vi "Rolling Average.vi"(7 "Enum":enum16{"Positive Slope", "Negative Slope"}(ring), 10 "Filtered X":dbl[](array[numeric]), 11 "Subset Length":i32) -> (3 "Averaged Values":dbl[][](array[numeric]))   [LabVIEW 2018]
uses:
  <vilib>/Analysis/baseanly.llb/Mean (DBL).vi
  <vilib>/Analysis/NI_AALBase.lvlib
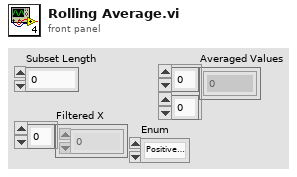
[diagram p1: front panel]
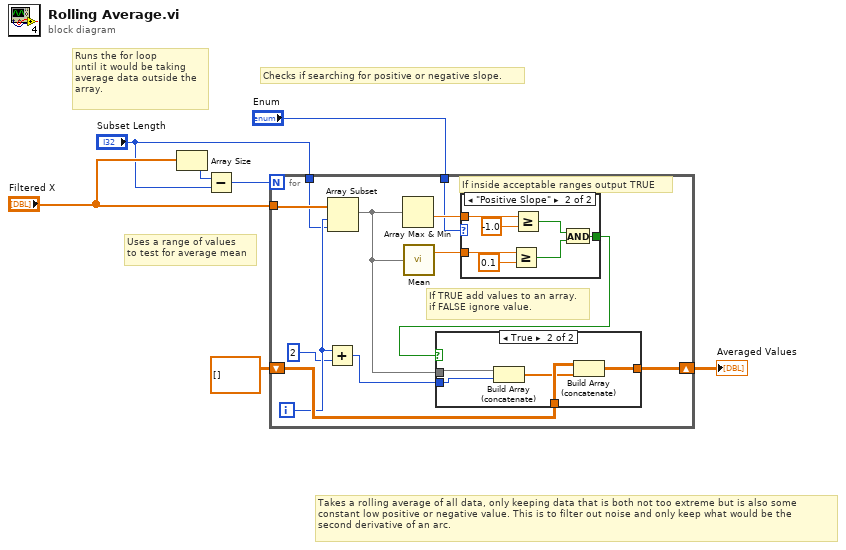
[diagram p0: block diagram]
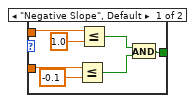
[diagram p2: hidden frame]
diagram:
  # "Uses a range of values\nto test for average mean"
  # "Checks if searching for positive or negative slope."
  # "Runs the for loop\nuntil it would be taking \naverage data outside the \narray."
  # "Takes a rolling average of all data, only keeping data that is both not too extreme but is also some\nconstant low positive or negative value. This is to filter out noise and only keep what would be the \nsecond derivative of an arc."
  n1 = Array Size(array="Filtered X") -> (size(s)=w3:i32)
  n2 = Subtract(x=w3, y="Subset Length") -> (x-y=w4:i32)
  n3 = for {
    N: w4 -> [_]
    tunnel: "Filtered X" -> [w19]
    shift-right: [w15] -> w7
    shift-left: dbl[][] [] -> [w14]
    tunnel: "Subset Length" -> [w10]
    tunnel: "Enum" -> [w9]
    i -> [w13]
    # "If TRUE add values to an array.\nif FALSE ignore value."
    # "If inside acceptable ranges output TRUE"
    n4 = Add(x=w13, y=2) -> (x+y=w11:i32)
    n5 = Array Subset(array=w19, index=w13, length=w10) -> (w16:dbl[])
    n6 = Array Max & Min(array=w16) -> (min value=w18:dbl)  [unwired: 3 out]
    n7 = call-poly <vilib>:"Mean.vi"("X"=w16) -> ("mean"=w17:dbl)  [unwired: 1 out]
    n8 = case shown="\"Positive Slope\"" w9 {
      tunnel: w18 -> [w22 w33]
      tunnel: w17 -> [w21 w31]
      tunnel: [w20 w27] -> w8
      frame "Negative Slope", Default {
        n9 = Less Or Equal?(x=w21, y=-0.1) -> (x <= y?=w23:bool)
        n10 = Less Or Equal?(x=w22, y=1.0) -> (x <= y?=w24:bool)
        n11 = And(x=w24, y=w23) -> (x .and. y?=w20:bool)
      }
      frame "Positive Slope" {
        n12 = Greater Or Equal?(x=w31, y=0.1) -> (x >= y?=w28:bool)
        n13 = Greater Or Equal?(x=w33, y=-1.0) -> (x >= y?=w29:bool)
        n14 = And(x=w29, y=w28) -> (x .and. y?=w27:bool)
      }
    }
    n15 = case shown="True" w8 {
      tunnel: w16 -> [_ w37]
      tunnel: [w34 w39] -> w15
      tunnel: w14 -> [w34 w38]
      tunnel: w11 -> [_ w36]
      frame False {
      }
      frame True {
        n16 = Build Array (concatenate)(w37, w36) -> (w35:dbl[])
        n17 = Build Array (concatenate)(w38, w35) -> (w39:dbl[][])
      }
    }
  }
  "Averaged Values" <- w7
